vi "Diode Current to Integer.vi"(10 "Max Current (mA)":dbl, 11 "Current (mA)":dbl) -> (3 "Current Int":i16)   [LabVIEW 2016, in "Laser Diode Controller.lvlib" / "KLD101.lvclass"]
uses:
  KLD101.lvclass
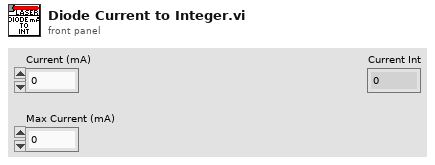
[diagram p1: front panel]
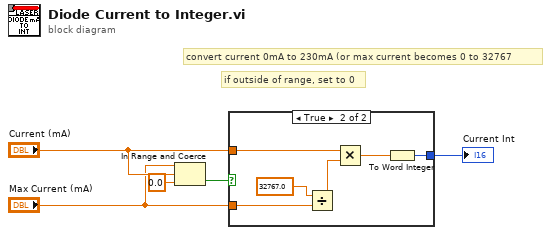
[diagram p0: block diagram]
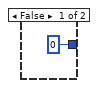
[diagram p2: hidden frame]
diagram:
  # "if outside of range, set to 0"
  # "convert current 0mA to 230mA (or max current becomes 0 to 32767"
  n1 = In Range and Coerce(upper limit="Max Current (mA)", x="Current (mA)", lower limit=0.0) -> (In Range?=w2:bool)  [unwired: 1 out]
  n2 = case shown="True" w2 {
    tunnel: [i16 0 w10] -> w5
    tunnel: "Current (mA)" -> [_ w9]
    tunnel: "Max Current (mA)" -> [_ w7]
    frame False {
    }
    frame True {
      n3 = Divide(x=32767.0 ("y"), y=w7) -> (x/y=w12:dbl)
      n4 = Multiply(x=w9, y=w12) -> (x*y=w8:dbl)
      n5 = To Word Integer(number=w8) -> (16bit integer=w10:i16)
    }
  }
  "Current Int" <- w5
